vi "LogFormatString.vi"(10 "Waveform Specification":T1, 11 "Timestamp":timestamp) -> (3 "resulting string":string)   [LabVIEW 2017, in "WaveformGenerator.lvlib"]
uses:
  WaveformGenerator.lvlib
  WaveformSpecs.ctl
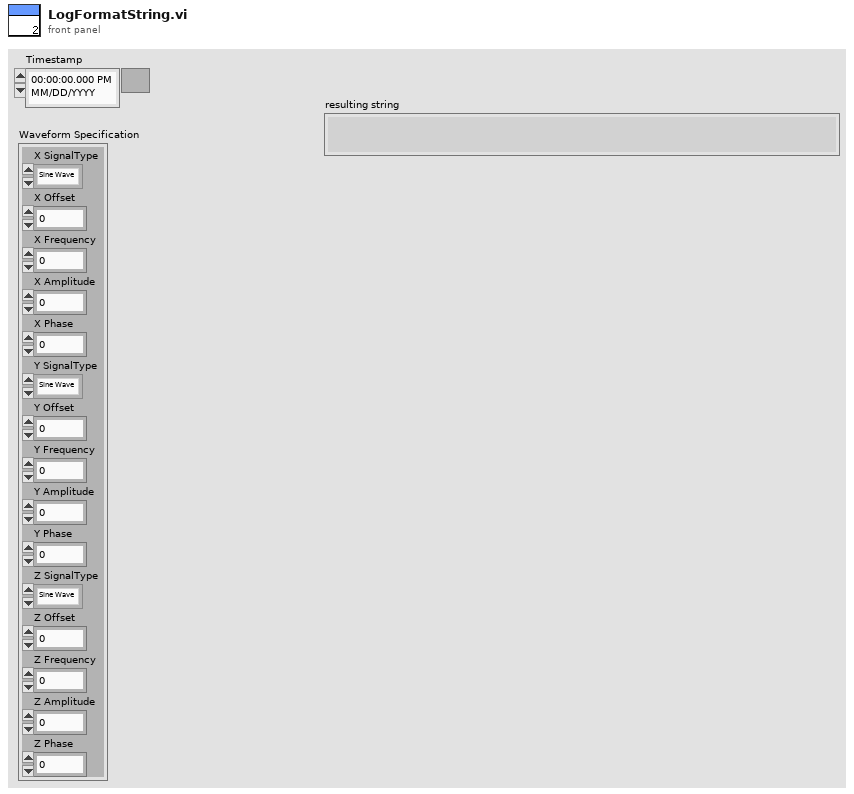
[diagram p1: front panel]
types:
  T1 = typedef "WaveformGenerator.lvlib/WaveformSpecs.ctl" = cluster{"X SignalType":enum16{"Sine Wave", "Triangle Wave", "Square Wave", "Sawtooth Wave"}, "X Offset":dbl, "X Frequency":dbl, "X Amplitude":dbl, "X Phase":dbl, "Y SignalType":enum16{"Sine Wave", "Triangle Wave", "Square Wave", "Sawtooth Wave"}, "Y Offset":dbl, "Y Frequency":dbl, "Y Amplitude":dbl, "Y Phase":dbl, "Z SignalType":enum16{"Sine Wave", "Triangle Wave", "Square Wave", "Sawtooth Wave"}, "Z Offset":dbl, "Z Frequency":dbl, "Z Amplitude":dbl, "Z Phase":dbl}
  T2 = enum16{"Sine Wave", "Triangle Wave", "Square Wave", "Sawtooth Wave"}
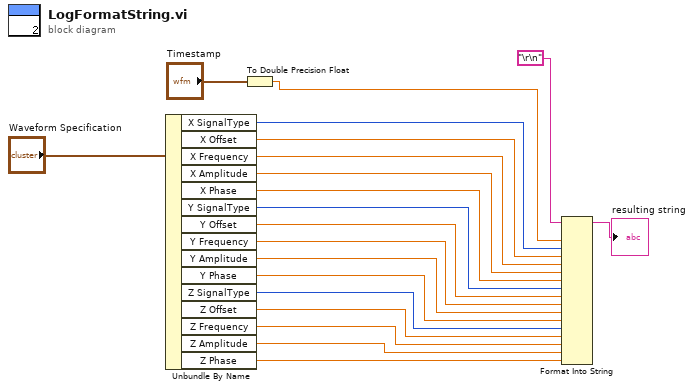
[diagram p0: block diagram]
diagram:
  n1 = Unbundle By Name("Waveform Specification") -> ("X SignalType"=w17:T2, "X Offset"=w16:dbl, "X Frequency"=w15:dbl, "X Amplitude"=w14:dbl, "X Phase"=w13:dbl, "Y SignalType"=w12:T2, "Y Offset"=w11:dbl, "Y Frequency"=w10:dbl, "Y Amplitude"=w9:dbl, "Y Phase"=w8:dbl, "Z SignalType"=w7:T2, "Z Offset"=w6:dbl, "Z Frequency"=w5:dbl, "Z Amplitude"=w4:dbl, "Z Phase"=w18:dbl)
  n2 = To Double Precision Float(number="Timestamp") -> (double precision float=w1:dbl)
  n3 = Format Into String(initial string="\r\n", w1, w17, w16, w15, w14, w13, w12, w11, w10, w9, w8, w7, w6, w5, w4, w18) -> (resulting string=→"resulting string":string)  [unwired: 2 in, 1 out]
